vi "svx_Waterfall Init.vi"(3 "Container State":T7={"Indicator?"=TRUE, "Run Mode?"=FALSE, " Refnum"=refnum}, 4 "Previous State":variant=variant(cluster{"X Scale Width %":dbl, "Y Scale Height %":dbl, "X-Axis Range":cluster{"Minimum":dbl, "Maximum":dbl}, "Y-Axis Range":cluster{"Minimum":dbl, "Maximum":dbl}, "Z-Axis Range":cluster{"Minimum":dbl, "Maximum":dbl}, "Plot Color":u32, "Frame Color":u32, "Background Color":u32, "Initial AutoScale Y":bool, "AutoScale X":u8, "AutoScale Y":u8, "AutoScale Z":u8, "Plot Transparency":bool, "X-Axis Name":string, "Y-Axis Name":string, "Z-Axis Name":string, "X-Axis Scaling Factor":cluster{"Offset":dbl, "Multiplier":dbl}, "Y-Axis Scaling Factor":cluster{"Offset":dbl, "Multiplier":dbl}, "Z-Axis Scaling Factor":cluster{"Offset":dbl, "Multiplier":dbl}, "X-Scale Visible":bool, "Y-Scale Visible":bool, "Z-Scale Visible":bool, "X-Scale Label Visible":bool, "Y-Scale Label Visible":bool, "Z-Scale Label Visible":bool, "X-Axis Range Scaled":cluster{"Minimum":dbl, "Maximum":dbl}, "Y-Axis Range Scaled":cluster{"Minimum":dbl, "Maximum":dbl}, "Z-Axis Range Scaled":cluster{"Minimum":dbl, "Maximum":dbl}, "Rev Z Order":bool, "X-Scale Format Str":string, "Y-Scale Format Str":string, "Z-Scale Format Str":string, "Decor color":u32, "Scale Range Change":refnum<user-event>, "out of state queue":refnum<queue>, "property nodes":refnum<queue>, "Lines":cluster{"Waterfall Cursor Line":cluster{"X":dbl, "Y":dbl, "Plot Number":i32}[]}[]} {"X Scale Width %"=80.4177545691906, "Y Scale Height %"=64.74820143884892, "X-Axis Range"={"Minimum"=0.0, "Maximum"=26000.0}, "Y-Axis Range"={"Minimum"=-60.0, "Maximum"=0.0}, "Z-Axis Range"={"Minimum"=0.0, "Maximum"=19.0}, "Plot Color"=61212, "Frame Color"=16252785, "Background Color"=16777222, "Initial AutoScale Y"=TRUE, "AutoScale X"=0, "AutoScale Y"=0, "AutoScale Z"=0, "Plot Transparency"=FALSE, "X-Axis Name"="Frequency", "Y-Axis Name"="Amplitude", "Z-Axis Name"="", "X-Axis Scaling Factor"={"Offset"=0.0, "Multiplier"=1.0}, "Y-Axis Scaling Factor"={"Offset"=0.0, "Multiplier"=1.0}, "Z-Axis Scaling Factor"={"Offset"=0.0, "Multiplier"=1.0}, "X-Scale Visible"=TRUE, "Y-Scale Visible"=TRUE, "Z-Scale Visible"=TRUE, "X-Scale Label Visible"=TRUE, "Y-Scale Label Visible"=TRUE, "Z-Scale Label Visible"=TRUE, "X-Axis Range Scaled"={"Minimum"=0.0, "Maximum"=26000.0}, "Y-Axis Range Scaled"={"Minimum"=-60.0, "Maximum"=0.0}, "Z-Axis Range Scaled"={"Minimum"=0.0, "Maximum"=19.0}, "Rev Z Order"=FALSE, "X-Scale Format Str"="%#.4g", "Y-Scale Format Str"="%#.4g", "Z-Scale Format Str"="%#.4g", "Decor color"=12369084, "Scale Range Change"=refnum, "out of state queue"=refnum, "property nodes"=refnum, "Lines"=[{"Waterfall Cursor Line"=[{"X"=0.0, "Y"=-10.306036706393398, "Plot Number"=0}, {"X"=4627.564263195183, "Y"=-4.153637411799666, "Plot Number"=1}, {"X"=7334.515826841692, "Y"=-3.5499069368758294, "Plot Number"=2}, {"X"=9255.128526390366, "Y"=-3.0722379606955927, "Plot Number"=3}, {"X"=10744.871473609634, "Y"=-3.0627425430263298, "Plot Number"=4}, {"X"=11962.080090036876, "Y"=-3.3477284130639164, "Plot Number"=5}, {"X"=12991.215311418866, "Y"=-3.1848657871720842, "Plot Number"=6}, {"X"=13882.69278958555, "Y"=-3.6843271671817974, "Plot Number"=7}, {"X"=14669.031653683383, "Y"=-3.821207941480867, "Plot Number"=8}, {"X"=15372.435736804815, "Y"=-4.143230158402616, "Plot Number"=9}, {"X"=16008.742129373426, "Y"=-3.1928926718910544, "Plot Number"=10}, {"X"=16589.64435323206, "Y"=-3.247711198602881, "Plot Number"=11}, {"X"=17124.022597777774, "Y"=-4.3178626545138945, "Plot Number"=12}, {"X"=17618.77957461405, "Y"=-3.8078221582138134, "Plot Number"=13}, {"X"=18079.387300451326, "Y"=-3.9782824916358455, "Plot Number"=14}, {"X"=18510.257052780733, "Y"=-3.243790976985388, "Plot Number"=15}, {"X"=18914.99697130832, "Y"=-3.5161678301773778, "Plot Number"=16}, {"X"=19296.595916878567, "Y"=-3.0414418556912164, "Plot Number"=17}, {"X"=19657.557553855113, "Y"=-3.142312605846323, "Plot Number"=18}, {"X"=20000.0, "Y"=-3.01005179578332, "Plot Number"=19}]}]}), 5 "Previous Version":T6={"Major"=10, "Minor"=0, "Fix"=0, "Build"=0}) -> (2 "Current State":T4={"X Scale Width %"=50.0, "Y Scale Height %"=50.0, "X-Axis Range"={"Minimum"=0.0, "Maximum"=10.0}, "Y-Axis Range"={"Minimum"=0.0, "Maximum"=10.0}, "Z-Axis Range"={"Minimum"=0.0, "Maximum"=10.0}, "Plot Color"=61212, "Frame Color"=16252785, "Background Color"=16777222, "Initial AutoScale Y"=TRUE, "AutoScale X"=2, "AutoScale Y"=2, "AutoScale Z"=2, "Plot Transparency"=FALSE, "X-Axis Name"="Frequency", "Y-Axis Name"="Amplitude", "Z-Axis Name"="", "X-Axis Scaling Factor"={"Offset"=0.0, "Multiplier"=1.0}, "Y-Axis Scaling Factor"={"Offset"=0.0, "Multiplier"=1.0}, "Z-Axis Scaling Factor"={"Offset"=0.0, "Multiplier"=1.0}, "X-Scale Visible"=TRUE, "Y-Scale Visible"=TRUE, "Z-Scale Visible"=TRUE, "X-Scale Label Visible"=TRUE, "Y-Scale Label Visible"=TRUE, "Z-Scale Label Visible"=TRUE, "X-Axis Range Scaled"={"Minimum"=0.0, "Maximum"=10.0}, "Y-Axis Range Scaled"={"Minimum"=0.0, "Maximum"=10.0}, "Z-Axis Range Scaled"={"Minimum"=0.0, "Maximum"=10.0}, "Rev Z Order"=FALSE, "X-Scale Format Str"="%#.4g", "Y-Scale Format Str"="%#.4g", "Z-Scale Format Str"="%#.4g", "Decor color"=12369084, "Scale Range Change"=refnum, "out of state queue"=refnum, "property nodes"=refnum, "Lines"=[], "Line Properties"={"Line Color"=61212, "Line Width"=61212, "Line Style"=enum."Dash", "DisplayLines"=FALSE}} {"Line Properties"."Line Width" min=1})   [LabVIEW 2017, in "SVX Waterfall Graph.xctl"]
uses:
  <vilib>/addons/_XControls/Waterfall Graph/SVX Waterfall Graph.xctl
  <vilib>/addons/_XControls/Waterfall Graph/subVIs/svx_Waterfall State.ctl
  <vilib>/addons/_NISVFA/_Shared subVIs/Controls/svc_Cluster of Array of Cluster of XYZ.ctl
  <vilib>/_xctls/Container State.ctl
  <vilib>/_xctls/Version.ctl
  <vilib>/_xctls/XControlSupport.lvlib
panel:
  in  "Indicator State (10.0.0.0)":T1={"X Scale Width %"=50.0, "Y Scale Height %"=50.0, "X-Axis Range"={"Minimum"=0.0, "Maximum"=10.0}, "Y-Axis Range"={"Minimum"=0.0, "Maximum"=10.0}, "Z-Axis Range"={"Minimum"=0.0, "Maximum"=10.0}, "Plot Color"=61212, "Frame Color"=16252785, "Background Color"=16777222, "Initial AutoScale Y"=TRUE, "AutoScale X"=2, "AutoScale Y"=2, "AutoScale Z"=2, "Plot Transparency"=FALSE, "X-Axis Name"="Frequency", "Y-Axis Name"="Amplitude", "Z-Axis Name"="", "X-Axis Scaling Factor"={"Offset"=0.0, "Multiplier"=1.0}, "Y-Axis Scaling Factor"={"Offset"=0.0, "Multiplier"=1.0}, "Z-Axis Scaling Factor"={"Offset"=0.0, "Multiplier"=1.0}, "X-Scale Visible"=TRUE, "Y-Scale Visible"=TRUE, "Z-Scale Visible"=TRUE, "X-Scale Label Visible"=TRUE, "Y-Scale Label Visible"=TRUE, "Z-Scale Label Visible"=TRUE, "X-Axis Range Scaled"={"Minimum"=0.0, "Maximum"=10.0}, "Y-Axis Range Scaled"={"Minimum"=0.0, "Maximum"=10.0}, "Z-Axis Range Scaled"={"Minimum"=0.0, "Maximum"=10.0}, "Rev Z Order"=FALSE, "X-Scale Format Str"="%#.4g", "Y-Scale Format Str"="%#.4g", "Z-Scale Format Str"="%#.4g", "Decor color"=12369084, "Scale Range Change"=refnum, "out of state queue"=refnum, "property nodes"=refnum}
  out "background":bool
  in  "Indicator State (6.0.0.0)":T2={"X Scale Width %"=80.0, "Y Scale Height %"=40.0, "X-Axis Range"={"Minimum"=0.0, "Maximum"=10.0}, "Y-Axis Range"={"Minimum"=0.0, "Maximum"=10.0}, "Z-Axis Range"={"Minimum"=0.0, "Maximum"=10.0}, "# Plots Updated"=0, "Plot Color"=61212, "Frame Color"=16252785, "Background Color"=16777222, "Property Name"=[], "Just Loaded?"=TRUE, "Initial AutoScale Y"=TRUE, "AutoScale X"=2, "AutoScale Y"=2, "AutoScale Z"=2, "Plot Transparency"=FALSE, "X-Axis Name"="Frequency", "Y-Axis Name"="Amplitude", "Z-Axis Name"="", "X-Axis Scaling Factor"={"Offset"=0.0, "Multiplier"=1.0}, "Y-Axis Scaling Factor"={"Offset"=0.0, "Multiplier"=1.0}, "Z-Axis Scaling Factor"={"Offset"=0.0, "Multiplier"=1.0}, "X-Scale Visible"=TRUE, "Y-Scale Visible"=TRUE, "Z-Scale Visible"=TRUE, "X-Scale Label Visible"=TRUE, "Y-Scale Label Visible"=TRUE, "Z-Scale Label Visible"=TRUE, "X-Axis Range Scaled"={"Minimum"=0.0, "Maximum"=10.0}, "Y-Axis Range Scaled"={"Minimum"=0.0, "Maximum"=10.0}, "Z-Axis Range Scaled"={"Minimum"=0.0, "Maximum"=10.0}, "Rev Z Order"=FALSE, "First Time Ever"=TRUE, "X-Scale Format Str"="%#.4g", "Y-Scale Format Str"="%#.4g", "Z-Scale Format Str"="%#.4g", "Decor color"=12369084, "Facade VI"=refnum, "Scale Range Change"=refnum}
  in  "Indicator State (5.0.0.0)":T3={"X Scale Width %"=80.0, "Y Scale Height %"=40.0, "X-Axis Range"={"Minimum"=0.0, "Maximum"=10.0}, "Y-Axis Range"={"Minimum"=0.0, "Maximum"=10.0}, "Z-Axis Range"={"Minimum"=0.0, "Maximum"=10.0}, "# Plots Updated"=0, "Plot Color"=61212, "Frame Color"=16252785, "Background Color"=16777222, "Property Name"=[], "Just Loaded?"=TRUE, "Initial AutoScale Y"=TRUE, "AutoScale X"=2, "AutoScale Y"=2, "AutoScale Z"=2, "Plot Transparency"=FALSE, "X-Axis Name"="Frequency", "Y-Axis Name"="Amplitude", "Z-Axis Name"="", "X-Axis Scaling Factor"={"Offset"=0.0, "Multiplier"=1.0}, "Y-Axis Scaling Factor"={"Offset"=0.0, "Multiplier"=1.0}, "Z-Axis Scaling Factor"={"Offset"=0.0, "Multiplier"=1.0}, "X-Scale Visible"=TRUE, "Y-Scale Visible"=TRUE, "Z-Scale Visible"=TRUE, "X-Scale Label Visible"=TRUE, "Y-Scale Label Visible"=TRUE, "Z-Scale Label Visible"=TRUE, "X-Axis Range Scaled"={"Minimum"=0.0, "Maximum"=10.0}, "Y-Axis Range Scaled"={"Minimum"=0.0, "Maximum"=10.0}, "Z-Axis Range Scaled"={"Minimum"=0.0, "Maximum"=10.0}, "Rev Z Order"=FALSE, "First Time Ever"=TRUE, "X-Scale Format Str"="%#.4g", "Y-Scale Format Str"="%#.4g", "Z-Scale Format Str"="%#.4g", "Decor color"=12369084, "Facade VI"=refnum}
  in  "Default Indicator State":T4={"X Scale Width %"=50.0, "Y Scale Height %"=50.0, "X-Axis Range"={"Minimum"=0.0, "Maximum"=10.0}, "Y-Axis Range"={"Minimum"=0.0, "Maximum"=10.0}, "Z-Axis Range"={"Minimum"=0.0, "Maximum"=10.0}, "Plot Color"=61212, "Frame Color"=16252785, "Background Color"=16777222, "Initial AutoScale Y"=TRUE, "AutoScale X"=2, "AutoScale Y"=2, "AutoScale Z"=2, "Plot Transparency"=FALSE, "X-Axis Name"="Frequency", "Y-Axis Name"="Amplitude", "Z-Axis Name"="", "X-Axis Scaling Factor"={"Offset"=0.0, "Multiplier"=1.0}, "Y-Axis Scaling Factor"={"Offset"=0.0, "Multiplier"=1.0}, "Z-Axis Scaling Factor"={"Offset"=0.0, "Multiplier"=1.0}, "X-Scale Visible"=TRUE, "Y-Scale Visible"=TRUE, "Z-Scale Visible"=TRUE, "X-Scale Label Visible"=TRUE, "Y-Scale Label Visible"=TRUE, "Z-Scale Label Visible"=TRUE, "X-Axis Range Scaled"={"Minimum"=0.0, "Maximum"=10.0}, "Y-Axis Range Scaled"={"Minimum"=0.0, "Maximum"=10.0}, "Z-Axis Range Scaled"={"Minimum"=0.0, "Maximum"=10.0}, "Rev Z Order"=FALSE, "X-Scale Format Str"="%#.4g", "Y-Scale Format Str"="%#.4g", "Z-Scale Format Str"="%#.4g", "Decor color"=12369084, "Scale Range Change"=refnum, "out of state queue"=refnum, "property nodes"=refnum, "Lines"=[], "Line Properties"={"Line Color"=16711680, "Line Width"=1, "Line Style"=enum."Solid", "DisplayLines"=TRUE}} {"Line Properties"."Line Width" min=1}
  in  "Default Control State":T4={"X Scale Width %"=50.0, "Y Scale Height %"=50.0, "X-Axis Range"={"Minimum"=0.0, "Maximum"=10.0}, "Y-Axis Range"={"Minimum"=0.0, "Maximum"=10.0}, "Z-Axis Range"={"Minimum"=0.0, "Maximum"=10.0}, "Plot Color"=61212, "Frame Color"=16252785, "Background Color"=16777222, "Initial AutoScale Y"=TRUE, "AutoScale X"=2, "AutoScale Y"=2, "AutoScale Z"=2, "Plot Transparency"=FALSE, "X-Axis Name"="Frequency", "Y-Axis Name"="Amplitude", "Z-Axis Name"="", "X-Axis Scaling Factor"={"Offset"=0.0, "Multiplier"=1.0}, "Y-Axis Scaling Factor"={"Offset"=0.0, "Multiplier"=1.0}, "Z-Axis Scaling Factor"={"Offset"=0.0, "Multiplier"=1.0}, "X-Scale Visible"=TRUE, "Y-Scale Visible"=TRUE, "Z-Scale Visible"=TRUE, "X-Scale Label Visible"=TRUE, "Y-Scale Label Visible"=TRUE, "Z-Scale Label Visible"=TRUE, "X-Axis Range Scaled"={"Minimum"=0.0, "Maximum"=10.0}, "Y-Axis Range Scaled"={"Minimum"=0.0, "Maximum"=10.0}, "Z-Axis Range Scaled"={"Minimum"=0.0, "Maximum"=10.0}, "Rev Z Order"=FALSE, "X-Scale Format Str"="%#.4g", "Y-Scale Format Str"="%#.4g", "Z-Scale Format Str"="%#.4g", "Decor color"=12369084, "Scale Range Change"=refnum, "out of state queue"=refnum, "property nodes"=refnum, "Lines"=[], "Line Properties"={"Line Color"=16711680, "Line Width"=1, "Line Style"=enum."Solid", "DisplayLines"=TRUE}} {"Line Properties"."Line Width" min=1}
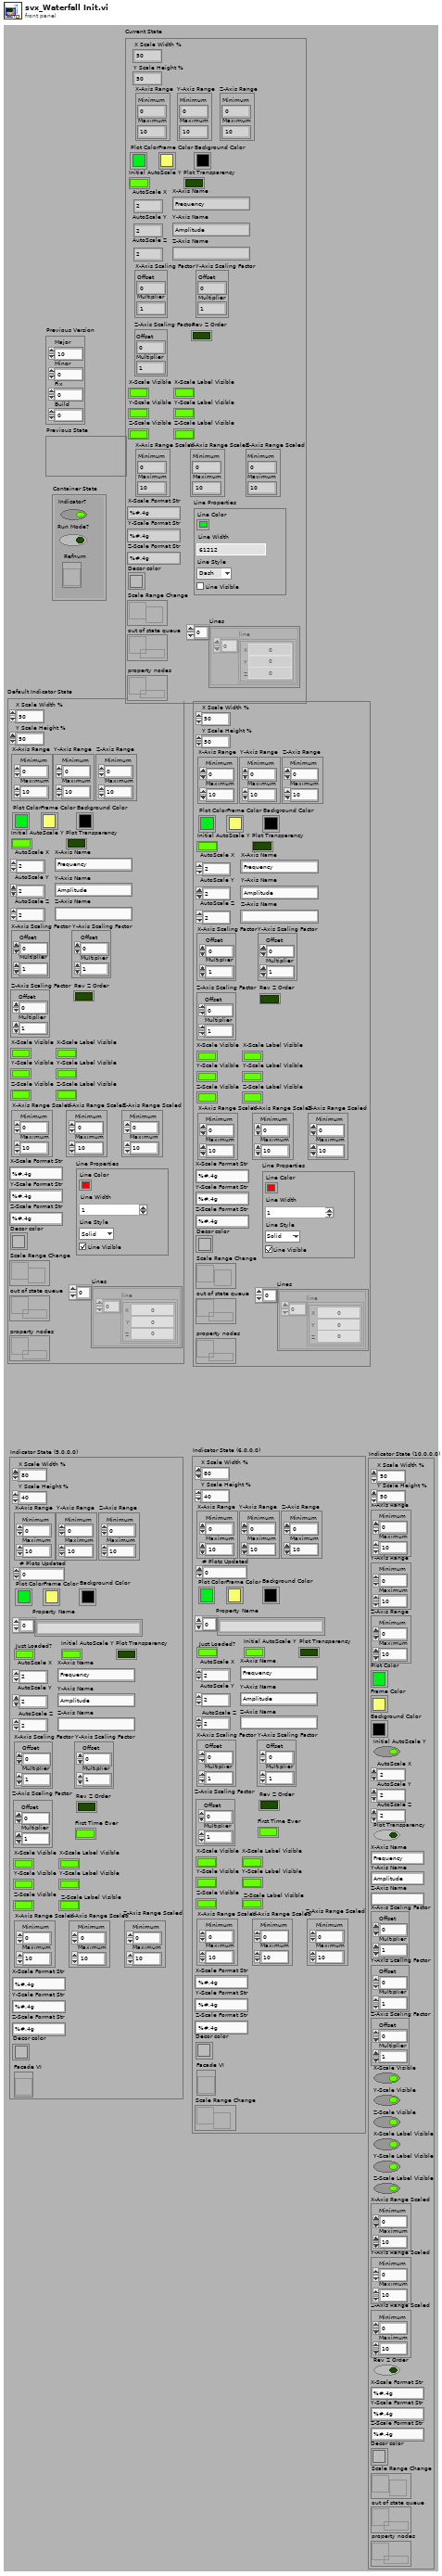
[diagram p1: front panel]
types:
  T1 = cluster{"X Scale Width %":dbl, "Y Scale Height %":dbl, "X-Axis Range":cluster{"Minimum":dbl, "Maximum":dbl}, "Y-Axis Range":cluster{"Minimum":dbl, "Maximum":dbl}, "Z-Axis Range":cluster{"Minimum":dbl, "Maximum":dbl}, "Plot Color":u32, "Frame Color":u32, "Background Color":u32, "Initial AutoScale Y":bool, "AutoScale X":u8, "AutoScale Y":u8, "AutoScale Z":u8, "Plot Transparency":bool, "X-Axis Name":string, "Y-Axis Name":string, "Z-Axis Name":string, "X-Axis Scaling Factor":cluster{"Offset":dbl, "Multiplier":dbl}, "Y-Axis Scaling Factor":cluster{"Offset":dbl, "Multiplier":dbl}, "Z-Axis Scaling Factor":cluster{"Offset":dbl, "Multiplier":dbl}, "X-Scale Visible":bool, "Y-Scale Visible":bool, "Z-Scale Visible":bool, "X-Scale Label Visible":bool, "Y-Scale Label Visible":bool, "Z-Scale Label Visible":bool, "X-Axis Range Scaled":cluster{"Minimum":dbl, "Maximum":dbl}, "Y-Axis Range Scaled":cluster{"Minimum":dbl, "Maximum":dbl}, "Z-Axis Range Scaled":cluster{"Minimum":dbl, "Maximum":dbl}, "Rev Z Order":bool, "X-Scale Format Str":string, "Y-Scale Format Str":string, "Z-Scale Format Str":string, "Decor color":u32, "Scale Range Change":refnum<user-event>, "out of state queue":refnum<queue>, "property nodes":refnum<queue>}
  T2 = cluster{"X Scale Width %":dbl, "Y Scale Height %":dbl, "X-Axis Range":cluster{"Minimum":dbl, "Maximum":dbl}, "Y-Axis Range":cluster{"Minimum":dbl, "Maximum":dbl}, "Z-Axis Range":cluster{"Minimum":dbl, "Maximum":dbl}, "# Plots Updated":i32, "Plot Color":u32, "Frame Color":u32, "Background Color":u32, "Property Name":string[], "Just Loaded?":bool, "Initial AutoScale Y":bool, "AutoScale X":u8, "AutoScale Y":u8, "AutoScale Z":u8, "Plot Transparency":bool, "X-Axis Name":string, "Y-Axis Name":string, "Z-Axis Name":string, "X-Axis Scaling Factor":cluster{"Offset":dbl, "Multiplier":dbl}, "Y-Axis Scaling Factor":cluster{"Offset":dbl, "Multiplier":dbl}, "Z-Axis Scaling Factor":cluster{"Offset":dbl, "Multiplier":dbl}, "X-Scale Visible":bool, "Y-Scale Visible":bool, "Z-Scale Visible":bool, "X-Scale Label Visible":bool, "Y-Scale Label Visible":bool, "Z-Scale Label Visible":bool, "X-Axis Range Scaled":cluster{"Minimum":dbl, "Maximum":dbl}, "Y-Axis Range Scaled":cluster{"Minimum":dbl, "Maximum":dbl}, "Z-Axis Range Scaled":cluster{"Minimum":dbl, "Maximum":dbl}, "Rev Z Order":bool, "First Time Ever":bool, "X-Scale Format Str":string, "Y-Scale Format Str":string, "Z-Scale Format Str":string, "Decor color":u32, "Facade VI":refnum<vi>, "Scale Range Change":refnum<user-event>}
  T3 = cluster{"X Scale Width %":dbl, "Y Scale Height %":dbl, "X-Axis Range":cluster{"Minimum":dbl, "Maximum":dbl}, "Y-Axis Range":cluster{"Minimum":dbl, "Maximum":dbl}, "Z-Axis Range":cluster{"Minimum":dbl, "Maximum":dbl}, "# Plots Updated":i32, "Plot Color":u32, "Frame Color":u32, "Background Color":u32, "Property Name":string[], "Just Loaded?":bool, "Initial AutoScale Y":bool, "AutoScale X":u8, "AutoScale Y":u8, "AutoScale Z":u8, "Plot Transparency":bool, "X-Axis Name":string, "Y-Axis Name":string, "Z-Axis Name":string, "X-Axis Scaling Factor":cluster{"Offset":dbl, "Multiplier":dbl}, "Y-Axis Scaling Factor":cluster{"Offset":dbl, "Multiplier":dbl}, "Z-Axis Scaling Factor":cluster{"Offset":dbl, "Multiplier":dbl}, "X-Scale Visible":bool, "Y-Scale Visible":bool, "Z-Scale Visible":bool, "X-Scale Label Visible":bool, "Y-Scale Label Visible":bool, "Z-Scale Label Visible":bool, "X-Axis Range Scaled":cluster{"Minimum":dbl, "Maximum":dbl}, "Y-Axis Range Scaled":cluster{"Minimum":dbl, "Maximum":dbl}, "Z-Axis Range Scaled":cluster{"Minimum":dbl, "Maximum":dbl}, "Rev Z Order":bool, "First Time Ever":bool, "X-Scale Format Str":string, "Y-Scale Format Str":string, "Z-Scale Format Str":string, "Decor color":u32, "Facade VI":refnum<vi>}
  T4 = typedef "SVX Waterfall Graph.xctl/svx_Waterfall State.ctl" = cluster{"X Scale Width %":dbl, "Y Scale Height %":dbl, "X-Axis Range":cluster{"Minimum":dbl, "Maximum":dbl}, "Y-Axis Range":cluster{"Minimum":dbl, "Maximum":dbl}, "Z-Axis Range":cluster{"Minimum":dbl, "Maximum":dbl}, "Plot Color":u32, "Frame Color":u32, "Background Color":u32, "Initial AutoScale Y":bool, "AutoScale X":u8, "AutoScale Y":u8, "AutoScale Z":u8, "Plot Transparency":bool, "X-Axis Name":string, "Y-Axis Name":string, "Z-Axis Name":string, "X-Axis Scaling Factor":cluster{"Offset":dbl, "Multiplier":dbl}, "Y-Axis Scaling Factor":cluster{"Offset":dbl, "Multiplier":dbl}, "Z-Axis Scaling Factor":cluster{"Offset":dbl, "Multiplier":dbl}, "X-Scale Visible":bool, "Y-Scale Visible":bool, "Z-Scale Visible":bool, "X-Scale Label Visible":bool, "Y-Scale Label Visible":bool, "Z-Scale Label Visible":bool, "X-Axis Range Scaled":cluster{"Minimum":dbl, "Maximum":dbl}, "Y-Axis Range Scaled":cluster{"Minimum":dbl, "Maximum":dbl}, "Z-Axis Range Scaled":cluster{"Minimum":dbl, "Maximum":dbl}, "Rev Z Order":bool, "X-Scale Format Str":string, "Y-Scale Format Str":string, "Z-Scale Format Str":string, "Decor color":u32, "Scale Range Change":refnum<user-event>, "out of state queue":refnum<queue>, "property nodes":refnum<queue>, "Lines":T5[], "Line Properties":cluster{"Line Color":u32, "Line Width":u16, "Line Style":enum32{"Solid", "Dash", "Dot", "DashDot", "DashDotDot"}, "DisplayLines":bool}}
  T5 = typedef "svc_Cluster of Array of Cluster of XYZ.ctl" = cluster{"line":cluster{"X":dbl, "Y":dbl, "Z":dbl}[]}
  T6 = typedef "XControlSupport.lvlib/Version.ctl" = cluster{"Major":u16, "Minor":u16, "Fix":u16, "Build":u16}
  T7 = typedef "XControlSupport.lvlib/Container State.ctl" = cluster{"Indicator?":bool, "Run Mode?":bool, " Refnum":refnum<vi>}
  T8 = cluster{"Minimum":dbl, "Maximum":dbl, "Kind":enum16{"X-Scale", "Y-Scale", "Z-Scale"}}
  T9 = cluster{"Line Color":u32, "Line Width":u16, "Line Style":enum32{"Solid", "Dash", "Dot", "DashDot", "DashDotDot"}, "DisplayLines":bool}
  T10 = cluster{"use queue?":bool, "X-Axis Range":cluster{"Minimum":dbl, "Maximum":dbl}, "Y-Axis Range":cluster{"Minimum":dbl, "Maximum":dbl}, "Z-Axis Range":cluster{"Minimum":dbl, "Maximum":dbl}, "X-Axis Range Scaled":cluster{"Minimum":dbl, "Maximum":dbl}, "Y-Axis Range Scaled":cluster{"Minimum":dbl, "Maximum":dbl}, "Z-Axis Range Scaled":cluster{"Minimum":dbl, "Maximum":dbl}, "AutoScale X":u8, "AutoScale Y":u8, "AutoScale Z":u8, "background":refnum<vi>}
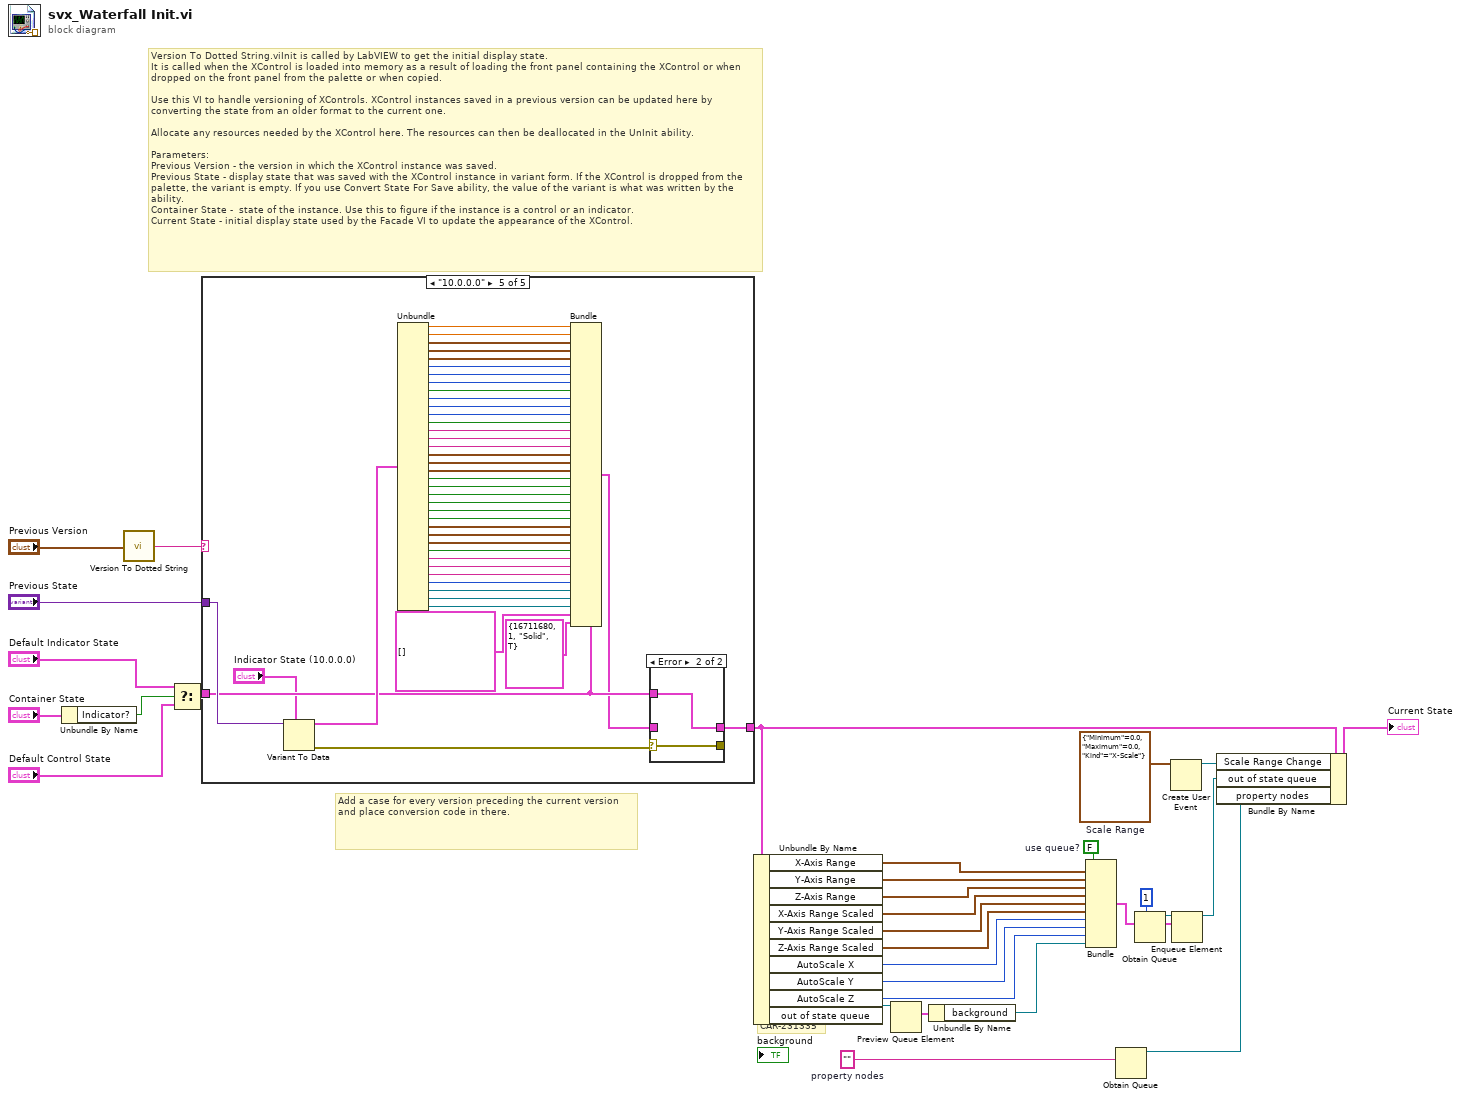
[diagram p0: block diagram]
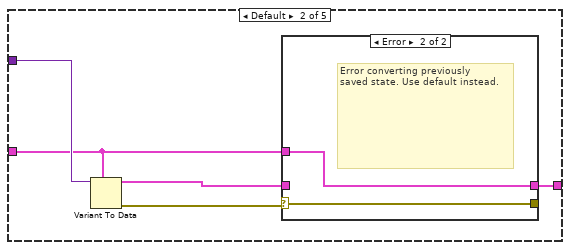
[diagram p3: hidden frame]
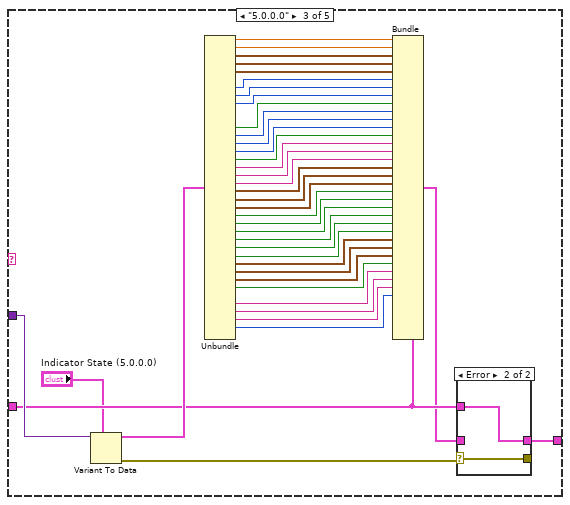
[diagram p5: hidden frame]
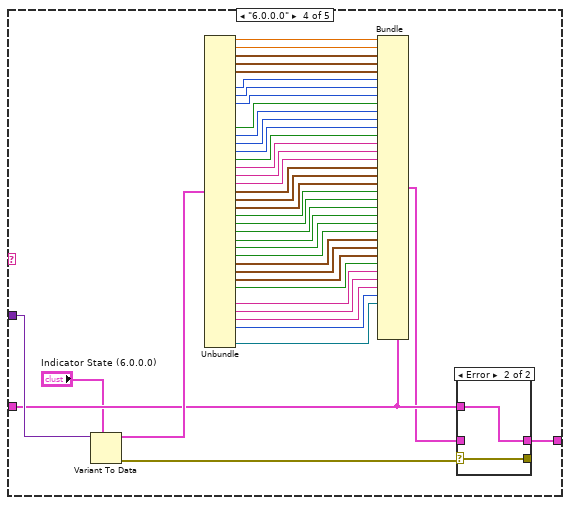
[diagram p7: hidden frame]
diagram:
  w20 = ""  # property nodes
  w12 = FALSE  # use queue?
  w22 = T8 {"Minimum"=0.0, "Maximum"=0.0, "Kind"=enum."X-Scale"}  # Scale Range
  # "CAR-231335"
  # "Add a case for every version preceding the current version and place conversion code in there."
  # "Version To Dotted String.viInit is called by LabVIEW to get the initial display state.\nIt is called when the XControl is loaded into memory as a result of loading the front panel containing the XControl or when dropped on the front panel from the palette or when copied.\n\nUse this VI to handle versioning of XControls. XControl instances saved in a previous version can be updated here by converting the state from an older format to the current one.\n\nAllocate any resources needed by the XControl here. The resources can then be deallocated in the UnInit ability.\n\nParameters:\nPrevious Version - the version in which the XControl instance was saved.\nPrevious State - display state that was saved with the XControl instance in variant form. If the XControl is dropped from the palette, the variant is empty. If you use Convert State For Save ability, the value of the variant is what was written by the ability. \nContainer State -  state of the instance. Use this to figure if the instance is a control or an indicator.\nCurrent State - initial display state used by the Facade VI to update the appearance of the XControl."
  n1 = Unbundle By Name("Container State") -> ("Indicator?"=w29:bool)
  n2 = call <vilib>:"Version To Dotted String.vi"("Version"="Previous Version") -> ("String Version"=w25:string)
  n3 = Select(t="Default Indicator State", s=w29, f="Default Control State") -> (s? t:f=w28:T4)
  n4 = case shown="\"10.0.0.0\"" w25 {
    tunnel: "Previous State" -> [_ w37 w81 w126 w175]
    tunnel: [w32 w34 w79 w124 w173] -> w8
    tunnel: w28 -> [w32 w35 w77 w122 w171]
    frame "0.0.0.0" {
      # "Just created, use default state"
    }
    frame Default {
      n5 = Variant To Data(type=w35, Variant=w37) -> (data=w33:T4, error out=w36:errorcluster)  [unwired: 1 in]
      n6 = case shown="Error" w36 {
        selector: w36 -> [w39 w40]
        tunnel: w33 -> [w38 _]
        tunnel: [w38 w41] -> w34
        tunnel: w35 -> [_ w41]
        tunnel: [w39 w40] -> _
        frame No Error {
        }
        frame Error {
          # "Error converting previously \nsaved state. Use default instead."
        }
      }
    }
    frame "5.0.0.0" {
      n7 = Variant To Data(type="Indicator State (5.0.0.0)", Variant=w81) -> (data=w78:T3, error out=w80:errorcluster)  [unwired: 1 in]
      n8 = Unbundle(w78) -> ("X Scale Width %"=w75:dbl, "Y Scale Height %"=w74:dbl, "X-Axis Range"=w73:cluster{"Minimum":dbl, "Maximum":dbl}, "Y-Axis Range"=w72:cluster{"Minimum":dbl, "Maximum":dbl}, "Z-Axis Range"=w71:cluster{"Minimum":dbl, "Maximum":dbl}, "Plot Color"=w69:u32, "Frame Color"=w68:u32, "Background Color"=w67:u32, "Initial AutoScale Y"=w66:bool, "AutoScale X"=w65:u8, "AutoScale Y"=w64:u8, "AutoScale Z"=w63:u8, "Plot Transparency"=w62:bool, "X-Axis Name"=w61:string, "Y-Axis Name"=w60:string, "Z-Axis Name"=w59:string, "X-Axis Scaling Factor"=w58:cluster{"Offset":dbl, "Multiplier":dbl}, "Y-Axis Scaling Factor"=w57:cluster{"Offset":dbl, "Multiplier":dbl}, "Z-Axis Scaling Factor"=w56:cluster{"Offset":dbl, "Multiplier":dbl}, "X-Scale Visible"=w55:bool, "Y-Scale Visible"=w54:bool, "Z-Scale Visible"=w53:bool, "X-Scale Label Visible"=w52:bool, "Y-Scale Label Visible"=w51:bool, "Z-Scale Label Visible"=w50:bool, "X-Axis Range Scaled"=w49:cluster{"Minimum":dbl, "Maximum":dbl}, "Y-Axis Range Scaled"=w48:cluster{"Minimum":dbl, "Maximum":dbl}, "Z-Axis Range Scaled"=w47:cluster{"Minimum":dbl, "Maximum":dbl}, "Rev Z Order"=w46:bool, "X-Scale Format Str"=w45:string, "Y-Scale Format Str"=w44:string, "Z-Scale Format Str"=w43:string, "Decor color"=w42:u32)  [unwired: 5 out]
      n9 = Bundle(cluster=w77, "X Scale Width %"=w75, "Y Scale Height %"=w74, "X-Axis Range"=w73, "Y-Axis Range"=w72, "Z-Axis Range"=w71, "Plot Color"=w69, "Frame Color"=w68, "Background Color"=w67, "Initial AutoScale Y"=w66, "AutoScale X"=w65, "AutoScale Y"=w64, "AutoScale Z"=w63, "Plot Transparency"=w62, "X-Axis Name"=w61, "Y-Axis Name"=w60, "Z-Axis Name"=w59, "X-Axis Scaling Factor"=w58, "Y-Axis Scaling Factor"=w57, "Z-Axis Scaling Factor"=w56, "X-Scale Visible"=w55, "Y-Scale Visible"=w54, "Z-Scale Visible"=w53, "X-Scale Label Visible"=w52, "Y-Scale Label Visible"=w51, "Z-Scale Label Visible"=w50, "X-Axis Range Scaled"=w49, "Y-Axis Range Scaled"=w48, "Z-Axis Range Scaled"=w47, "Rev Z Order"=w46, "X-Scale Format Str"=w45, "Y-Scale Format Str"=w44, "Z-Scale Format Str"=w43, "Decor color"=w42) -> (w70:T4)  [unwired: 5 in]
      n10 = case shown="Error" w80 {
        selector: w80 -> [w83 w84]
        tunnel: w70 -> [w82 _]
        tunnel: [w82 w85] -> w79
        tunnel: w77 -> [_ w85]
        tunnel: [w83 w84] -> _
        frame No Error {
        }
        frame Error {
        }
      }
    }
    frame "6.0.0.0" {
      n11 = Variant To Data(type="Indicator State (6.0.0.0)", Variant=w126) -> (data=w123:T2, error out=w125:errorcluster)  [unwired: 1 in]
      n12 = Unbundle(w123) -> ("X Scale Width %"=w120:dbl, "Y Scale Height %"=w119:dbl, "X-Axis Range"=w118:cluster{"Minimum":dbl, "Maximum":dbl}, "Y-Axis Range"=w117:cluster{"Minimum":dbl, "Maximum":dbl}, "Z-Axis Range"=w116:cluster{"Minimum":dbl, "Maximum":dbl}, "Plot Color"=w114:u32, "Frame Color"=w113:u32, "Background Color"=w112:u32, "Initial AutoScale Y"=w111:bool, "AutoScale X"=w110:u8, "AutoScale Y"=w109:u8, "AutoScale Z"=w108:u8, "Plot Transparency"=w107:bool, "X-Axis Name"=w106:string, "Y-Axis Name"=w105:string, "Z-Axis Name"=w104:string, "X-Axis Scaling Factor"=w103:cluster{"Offset":dbl, "Multiplier":dbl}, "Y-Axis Scaling Factor"=w102:cluster{"Offset":dbl, "Multiplier":dbl}, "Z-Axis Scaling Factor"=w101:cluster{"Offset":dbl, "Multiplier":dbl}, "X-Scale Visible"=w100:bool, "Y-Scale Visible"=w99:bool, "Z-Scale Visible"=w98:bool, "X-Scale Label Visible"=w97:bool, "Y-Scale Label Visible"=w96:bool, "Z-Scale Label Visible"=w95:bool, "X-Axis Range Scaled"=w94:cluster{"Minimum":dbl, "Maximum":dbl}, "Y-Axis Range Scaled"=w93:cluster{"Minimum":dbl, "Maximum":dbl}, "Z-Axis Range Scaled"=w92:cluster{"Minimum":dbl, "Maximum":dbl}, "Rev Z Order"=w91:bool, "X-Scale Format Str"=w90:string, "Y-Scale Format Str"=w89:string, "Z-Scale Format Str"=w88:string, "Decor color"=w87:u32, "Scale Range Change"=w86:refnum<user-event>)  [unwired: 5 out]
      n13 = Bundle(cluster=w122, "X Scale Width %"=w120, "Y Scale Height %"=w119, "X-Axis Range"=w118, "Y-Axis Range"=w117, "Z-Axis Range"=w116, "Plot Color"=w114, "Frame Color"=w113, "Background Color"=w112, "Initial AutoScale Y"=w111, "AutoScale X"=w110, "AutoScale Y"=w109, "AutoScale Z"=w108, "Plot Transparency"=w107, "X-Axis Name"=w106, "Y-Axis Name"=w105, "Z-Axis Name"=w104, "X-Axis Scaling Factor"=w103, "Y-Axis Scaling Factor"=w102, "Z-Axis Scaling Factor"=w101, "X-Scale Visible"=w100, "Y-Scale Visible"=w99, "Z-Scale Visible"=w98, "X-Scale Label Visible"=w97, "Y-Scale Label Visible"=w96, "Z-Scale Label Visible"=w95, "X-Axis Range Scaled"=w94, "Y-Axis Range Scaled"=w93, "Z-Axis Range Scaled"=w92, "Rev Z Order"=w91, "X-Scale Format Str"=w90, "Y-Scale Format Str"=w89, "Z-Scale Format Str"=w88, "Decor color"=w87, "Scale Range Change"=w86) -> (w115:T4)  [unwired: 4 in]
      n14 = case shown="Error" w125 {
        selector: w125 -> [w128 w129]
        tunnel: w115 -> [w127 _]
        tunnel: [w127 w130] -> w124
        tunnel: w122 -> [_ w130]
        tunnel: [w128 w129] -> _
        frame No Error {
        }
        frame Error {
        }
      }
    }
    frame "10.0.0.0" {
      n15 = Variant To Data(type="Indicator State (10.0.0.0)", Variant=w175) -> (data=w172:T1, error out=w174:errorcluster)  [unwired: 1 in]
      n16 = Unbundle(w172) -> ("X Scale Width %"=w170:dbl, "Y Scale Height %"=w169:dbl, "X-Axis Range"=w168:cluster{"Minimum":dbl, "Maximum":dbl}, "Y-Axis Range"=w167:cluster{"Minimum":dbl, "Maximum":dbl}, "Z-Axis Range"=w166:cluster{"Minimum":dbl, "Maximum":dbl}, "Plot Color"=w135:u32, "Frame Color"=w134:u32, "Background Color"=w133:u32, "Initial AutoScale Y"=w136:bool, "AutoScale X"=w137:u8, "AutoScale Y"=w138:u8, "AutoScale Z"=w139:u8, "Plot Transparency"=w140:bool, "X-Axis Name"=w141:string, "Y-Axis Name"=w142:string, "Z-Axis Name"=w143:string, "X-Axis Scaling Factor"=w144:cluster{"Offset":dbl, "Multiplier":dbl}, "Y-Axis Scaling Factor"=w145:cluster{"Offset":dbl, "Multiplier":dbl}, "Z-Axis Scaling Factor"=w146:cluster{"Offset":dbl, "Multiplier":dbl}, "X-Scale Visible"=w147:bool, "Y-Scale Visible"=w148:bool, "Z-Scale Visible"=w149:bool, "X-Scale Label Visible"=w150:bool, "Y-Scale Label Visible"=w151:bool, "Z-Scale Label Visible"=w152:bool, "X-Axis Range Scaled"=w153:cluster{"Minimum":dbl, "Maximum":dbl}, "Y-Axis Range Scaled"=w154:cluster{"Minimum":dbl, "Maximum":dbl}, "Z-Axis Range Scaled"=w155:cluster{"Minimum":dbl, "Maximum":dbl}, "Rev Z Order"=w156:bool, "X-Scale Format Str"=w159:string, "Y-Scale Format Str"=w158:string, "Z-Scale Format Str"=w157:string, "Decor color"=w163:u32, "Scale Range Change"=w162:refnum<user-event>, "out of state queue"=w161:refnum<queue>, "property nodes"=w160:refnum<queue>)
      n17 = Bundle(cluster=w171, "X Scale Width %"=w170, "Y Scale Height %"=w169, "X-Axis Range"=w168, "Y-Axis Range"=w167, "Z-Axis Range"=w166, "Plot Color"=w135, "Frame Color"=w134, "Background Color"=w133, "Initial AutoScale Y"=w136, "AutoScale X"=w137, "AutoScale Y"=w138, "AutoScale Z"=w139, "Plot Transparency"=w140, "X-Axis Name"=w141, "Y-Axis Name"=w142, "Z-Axis Name"=w143, "X-Axis Scaling Factor"=w144, "Y-Axis Scaling Factor"=w145, "Z-Axis Scaling Factor"=w146, "X-Scale Visible"=w147, "Y-Scale Visible"=w148, "Z-Scale Visible"=w149, "X-Scale Label Visible"=w150, "Y-Scale Label Visible"=w151, "Z-Scale Label Visible"=w152, "X-Axis Range Scaled"=w153, "Y-Axis Range Scaled"=w154, "Z-Axis Range Scaled"=w155, "Rev Z Order"=w156, "X-Scale Format Str"=w159, "Y-Scale Format Str"=w158, "Z-Scale Format Str"=w157, "Decor color"=w163, "Scale Range Change"=w162, "out of state queue"=w161, "property nodes"=w160, "Lines"=T5[] [], "Line Properties"=T9 {"Line Color"=16711680, "Line Width"=1, "Line Style"=enum."Solid", "DisplayLines"=TRUE}) -> (w165:T4)
      n18 = case shown="Error" w174 {
        selector: w174 -> [w177 w178]
        tunnel: w165 -> [w176 _]
        tunnel: [w176 w179] -> w173
        tunnel: w171 -> [_ w179]
        tunnel: [w177 w178] -> _
        frame No Error {
        }
        frame Error {
        }
      }
    }
  }
  n19 = Unbundle By Name(w8) -> ("X-Axis Range"=w10:cluster{"Minimum":dbl, "Maximum":dbl}, "Y-Axis Range"=w11:cluster{"Minimum":dbl, "Maximum":dbl}, "Z-Axis Range"=w15:cluster{"Minimum":dbl, "Maximum":dbl}, "X-Axis Range Scaled"=w16:cluster{"Minimum":dbl, "Maximum":dbl}, "Y-Axis Range Scaled"=w17:cluster{"Minimum":dbl, "Maximum":dbl}, "Z-Axis Range Scaled"=w18:cluster{"Minimum":dbl, "Maximum":dbl}, "AutoScale X"=w7:u8, "AutoScale Y"=w6:u8, "AutoScale Z"=w5:u8, "out of state queue"=w3:refnum<queue>)
  n20 = Preview Queue Element(queue=w3) -> (element=w2:T10)  [unwired: 2 in, 3 out]
  n21 = Unbundle By Name(w2) -> ("background"=w1:refnum<vi>)
  n22 = Bundle("use queue?"=w12, "X-Axis Range"=w10, "Y-Axis Range"=w11, "Z-Axis Range"=w15, "X-Axis Range Scaled"=w16, "Y-Axis Range Scaled"=w17, "Z-Axis Range Scaled"=w18, "AutoScale X"=w7, "AutoScale Y"=w6, "AutoScale Z"=w5, "background"=w1) -> (w14:T10)  [unwired: 1 in]
  n23 = Obtain Queue(element data type=w20) -> (queue out=w9:refnum<queue>)  [unwired: 4 in, 2 out]
  n24 = Obtain Queue(max queue size (-1, unlimited)=1, element data type=w14) -> (queue out=w19:refnum<queue>)  [unwired: 3 in, 2 out]
  n25 = Create User Event(user event datatype=w22) -> (user event=w23:refnum<user-event>)  [unwired: 1 in, 1 out]
  n26 = Enqueue Element(queue=w19, element=w14) -> (queue out=w4:refnum<queue>)  [unwired: 2 in, 2 out]
  n27 = Bundle By Name(cluster=w8, "Scale Range Change"=w23, "out of state queue"=w4, "property nodes"=w9) -> (→"Current State":T4)
